vi "Set Dialog Properties.vi"(8 "error in (no error)":errorcluster, 10 "Boolean":bool, 11 "VI in":refnum<vi>) -> (0 "error out":errorcluster, 3 "VI out":refnum<vi>)   [LabVIEW 2015]
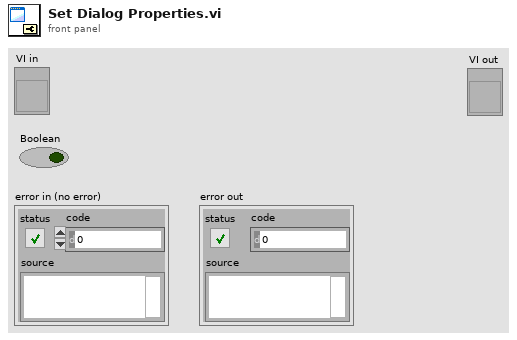
[diagram p1: front panel]
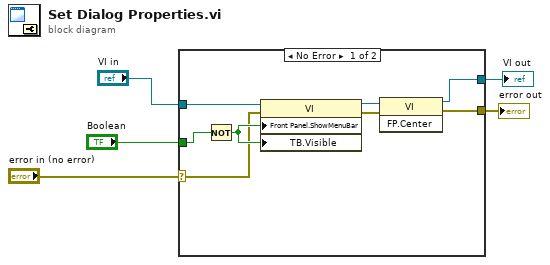
[diagram p0: block diagram]
diagram:
  n1 = case shown="No Error" "error in (no error)" {
    selector: "error in (no error)" -> [w6 w14]
    tunnel: [w13 w14] -> w5
    tunnel: "VI in" -> [w12 w15]
    tunnel: "Boolean" -> [w7 _]
    tunnel: [w9 w15] -> w1
    frame No Error {
      n2 = Not(x=w7) -> (.not. x?=w8:bool)
      n3 = property class="VI"(reference=w12, error in=w6, "Front Panel.ShowMenuBar"=w8, "TB.Visible"=w8) -> (reference out=w10:refnum<vi>, error out=w11:errorcluster)
      n4 = invoke class="VI" method="FP.Center"(reference=w10, error in=w11) -> (reference out=w9:refnum<vi>, error out=w13:errorcluster)  [unwired: 1 in, 1 out]
    }
    frame Error {
    }
  }
  "error out" <- w5
  "VI out" <- w1
